vi "Convert EngineeringUnits to RawVal.vi"(8 "error in (no error)":errorcluster, 9 "Coerce (false)?":bool, 10 "Engineering Units In":dbl format="%.3g", 11 "Conversion":T1 {"ScaleOffset" format="%.3f"; "MinEngUnit" format="%.3f"; "MaxEngUnit" format="%.3f"; "MinSignal" format="%.3f"; "MaxSignal" format="%.3f"}) -> (0 "error out":errorcluster, 1 "In Range?":bool, 2 "Raw Value Out":dbl format="%.3g")   [LabVIEW 2022 SP3, in "DAQ.lvclass"]
doc: "Developed by Kevin Thompson\nkevin@thompsonengineering.net\n\nCopyright 2018-2020\nThompson Engineering, LLC"
uses:
  DAQ.lvclass
  DataTypes/TD DataValueConversion--cluster.ctl
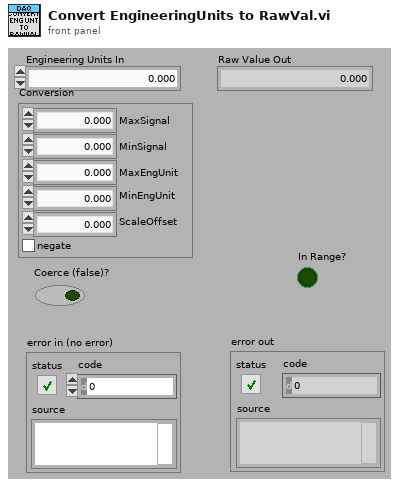
[diagram p1: front panel]
types:
  T1 = typedef "DAQ.lvclass/TD DataValueConversion--cluster.ctl" = cluster{"MaxSignal":dbl, "MinSignal":dbl, "MaxEngUnit":dbl, "MinEngUnit":dbl, "ScaleOffset":dbl, "negate":bool}
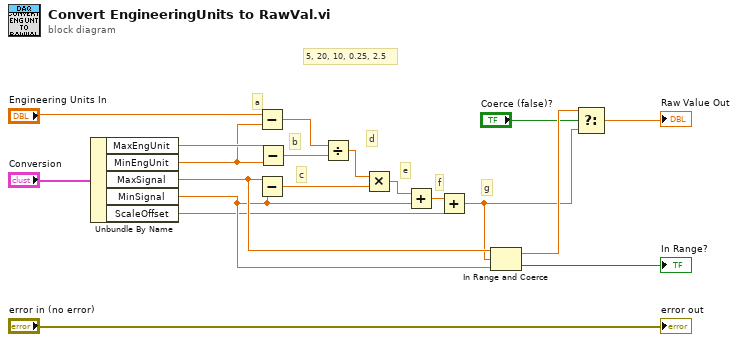
[diagram p0: block diagram]
diagram:
  # "5, 20, 10, 0.25, 2.5"
  # "g"
  # "f"
  # "e"
  # "d"
  # "c"
  # "b"
  # "a"
  n1 = Unbundle By Name("Conversion") -> ("MaxEngUnit"=w19:dbl, "MinEngUnit"=w18:dbl, "MaxSignal"=w9:dbl, "MinSignal"=w4:dbl, "ScaleOffset"=w2:dbl)
  n2 = Subtract(x="Engineering Units In", y=w18) -> (x-y=w17:dbl)
  n3 = Subtract(x=w9, y=w4) -> (x-y=w15:dbl)
  n4 = Subtract(x=w19, y=w18) -> (x-y=w16:dbl)
  n5 = Divide(x=w17, y=w16) -> (x/y=w14:dbl)
  n6 = Multiply(x=w14, y=w15) -> (x*y=w13:dbl)
  n7 = Add(x=w13, y=w4) -> (x+y=w3:dbl)
  n8 = Add(x=w3, y=w2) -> (x+y=w1:dbl)
  n9 = In Range and Coerce(upper limit=w9, x=w1, lower limit=w4) -> (coerced(x)=w8:dbl, In Range?=→"In Range?":bool)
  n10 = Select(t=w8, s="Coerce (false)?", f=w1) -> (s? t:f=→"Raw Value Out":dbl)
  "error out" <- "error in (no error)"
